vi "SetGXMLCfgRes.vi"(8 "error in (no error)":errorcluster, 10 "ResChanCfg":T1, 11 "Resistance in":refnum<class "Resistance.lvclass">) -> (0 "error out":errorcluster, 3 "Resistance out":refnum<class "Resistance.lvclass">)   [LabVIEW 2012, in "Measurement Channels.lvlib" / "Resistance.lvclass"]
uses:
  Resistance.lvclass
  ResProps_TD.ctl
  Resistance.lvclass/Resistance.ctl
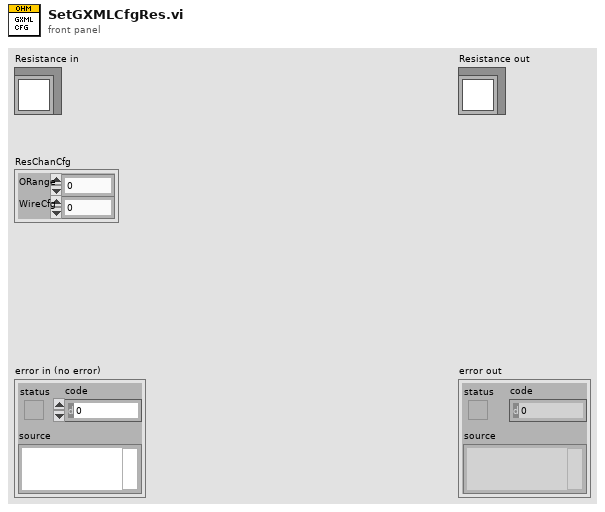
[diagram p1: front panel]
types:
  T1 = typedef "Measurement Channels.lvlib/Resistance.lvclass/ResProps_TD.ctl" = cluster{"ORange":u16, "WireCfg":u16}
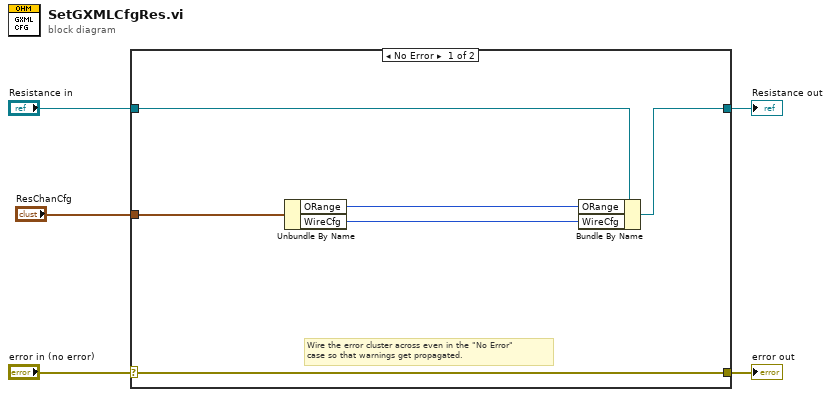
[diagram p0: block diagram]
diagram:
  n1 = case shown="No Error" "error in (no error)" {
    selector: "error in (no error)" -> [w11 w13]
    tunnel: [w11 w13] -> w4
    tunnel: [w6 w12] -> w2
    tunnel: "Resistance in" -> [w7 w12]
    tunnel: "ResChanCfg" -> [w8 _]
    frame No Error {
      # "Wire the error cluster across even in the \"No Error\"\ncase so that warnings get propagated."
      n2 = Unbundle By Name(w8) -> ("ORange"=w10:u16, "WireCfg"=w9:u16)
      n3 = Bundle By Name(cluster=w7, "ORange"=w10, "WireCfg"=w9) -> (w6:refnum<class "Resistance.lvclass">)
    }
    frame Error {
    }
  }
  "error out" <- w4
  "Resistance out" <- w2
